vi "WriteConfiguration.vi"(8 "error in":errorcluster) -> (0 "error out":errorcluster)   [LabVIEW 2013]
uses:
  GlobalVariables/ValveParameters.vi
  <vilib>/Utility/config.llb/Write Key (U32).vi
  <vilib>/Utility/config.llb/Write Key (String).vi
  <vilib>/Utility/config.llb/Write Key (I32).vi
  GlobalVariables/CaptParameters.vi
  GlobalVariables/SystemParameters.vi
  GlobalVariables/PreconfiguredSleeveData.vi
  GlobalVariables/LanguagesSettings.vi
  <vilib>/Utility/config.llb/NI_LVConfig.lvlib
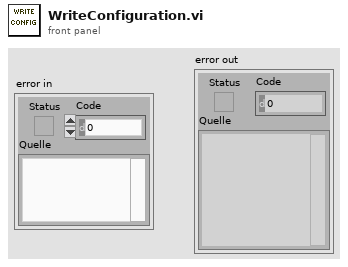
[diagram p1: front panel]
types:
  T1 = cluster{"baudrate":u32, "databits":u16, "paritybit":u16, "stopbits":u16, "flux control":u16, "Port":string, "Serial Parameters":cluster{"Mode":enum16{"RTU", "ASCII"}, "Slave Address":u8}, "Timeout":u32}
  T2 = typedef "NI_LVConfig.lvlib/Config Data RefNum.ctl" = refnum<k1>
  T3 = cluster{"baudrate":u32, "databits":u16, "paritybit":u16, "stopbits":u16, "flux control":u16, "Port":string, "Register Address":u16, "Serial Parameters":cluster{"Mode":enum16{"RTU", "ASCII"}, "Slave Address":u8}, "Timeout":u32}
  T4 = cluster{"defaultLanguage":string, "languageFile":string, "languages":string, "calibrationVolumeFile":string}
  T5 = cluster{"sleeveLength":dbl, "sleeveDiameter":dbl, "sleeveThickness":dbl}
  T6 = cluster{"SupportedLanguagesList":string[], "ActiveLanguage":string, "ActiveLanguageIndex":u16, "LocalisationFileContent[out]":cluster{"Indices":u32[], "LocalizedWords":string[][]}}
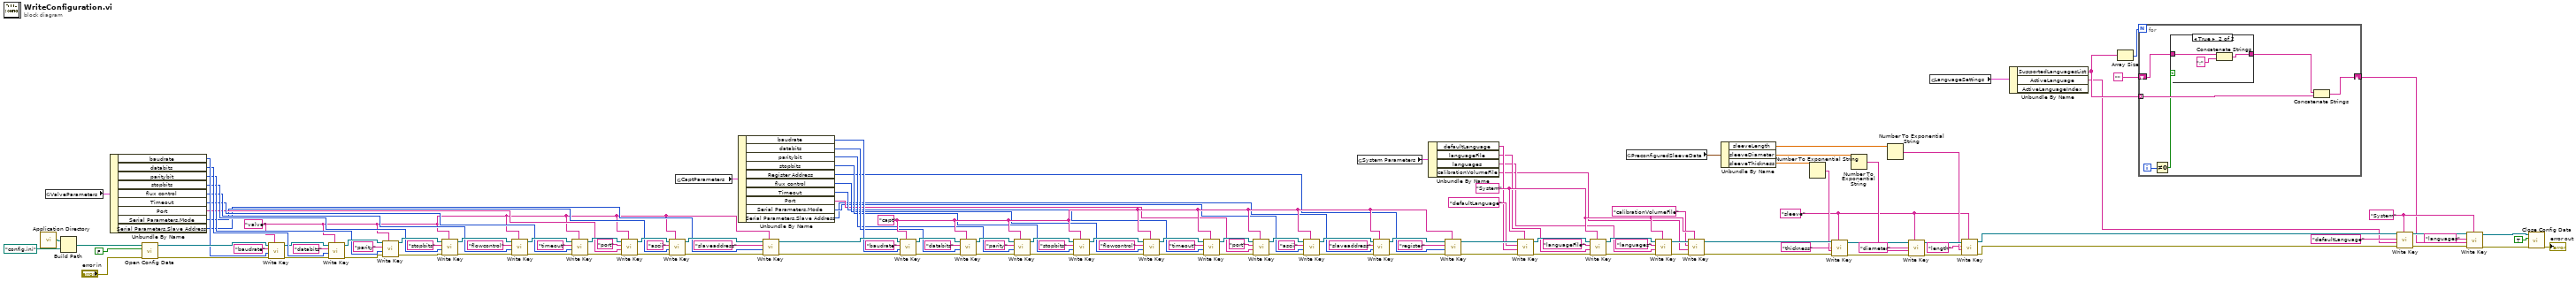
[diagram p0: block diagram]
diagram:
  w5 = "System"
  w19 = "sleeve"
  w41 = "System"
  w68 = "capt" ("section")
  w93 = "valve" ("section")
  n1 = call <vilib>:"Application Directory.vi"() -> ("Application Directory"=w130:path)
  n2 = global read "ValveParameters.vi" "ValveParameters"() -> (w127:T1)
  n3 = Build Path(base path=w130, name or relative path=path "config.ini" ("configuration file path")) -> (appended path=w128:path)
  n4 = Unbundle By Name(w127) -> ("baudrate"=w125:u32, "databits"=w122:u16, "paritybit"=w103:u16, "stopbits"=w102:u16, "flux control"=w101:u16, "Timeout"=w100:u32, "Port"=w99:string, "Serial Parameters.Mode"=w96:enum16{"RTU", "ASCII"}, "Serial Parameters.Slave Address"=w95:u8)
  n5 = call <vilib>:"Open Config Data.vi"("error in (no error)"="error in", "create file if necessary (T)"=FALSE ("create file if necessary? (T)"), "configuration file path"=w128) -> ("error out"=w137:errorcluster, "refnum"=w136:T2)  [unwired: 6 in, 1 out]
  n6 = call-poly <vilib>:"Write Key.vi"("section"=w93, "error in (no error)"=w137, "value"=w125, "key"="baudrate", "refnum"=w136) -> ("error out"=w134:errorcluster, "refnum out"=w121:T2)  [unwired: 4 in, 1 out]
  n7 = call-poly <vilib>:"Write Key.vi"("section"=w93, "error in (no error)"=w134, "value"=w122, "key"="databits", "refnum"=w121) -> ("error out"=w135:errorcluster, "refnum out"=w120:T2)  [unwired: 4 in, 1 out]
  n8 = call-poly <vilib>:"Write Key.vi"("section"=w93, "error in (no error)"=w135, "value"=w103, "key"="parity", "refnum"=w120) -> ("error out"=w114:errorcluster, "refnum out"=w119:T2)  [unwired: 4 in, 1 out]
  n9 = call-poly <vilib>:"Write Key.vi"("section"=w93, "error in (no error)"=w114, "value"=w102, "key"="stopbits", "refnum"=w119) -> ("error out"=w113:errorcluster, "refnum out"=w118:T2)  [unwired: 4 in, 1 out]
  n10 = call-poly <vilib>:"Write Key.vi"("section"=w93, "error in (no error)"=w113, "value"=w101, "key"="flowcontrol", "refnum"=w118) -> ("error out"=w112:errorcluster, "refnum out"=w117:T2)  [unwired: 4 in, 1 out]
  n11 = call-poly <vilib>:"Write Key.vi"("section"=w93, "error in (no error)"=w112, "value"=w100, "key"="timeout", "refnum"=w117) -> ("error out"=w111:errorcluster, "refnum out"=w116:T2)  [unwired: 4 in, 1 out]
  n12 = call-poly <vilib>:"Write Key.vi"("section"=w93, "error in (no error)"=w111, "value"=w99, "key"="port", "refnum"=w116) -> ("error out"=w110:errorcluster, "refnum out"=w115:T2)  [unwired: 4 in, 1 out]
  n13 = call-poly <vilib>:"Write Key.vi"("section"=w93, "error in (no error)"=w110, "value"=w96, "key"="ascii", "refnum"=w115) -> ("error out"=w109:errorcluster, "refnum out"=w108:T2)  [unwired: 4 in, 1 out]
  n14 = global read "CaptParameters.vi" "CaptParameters"() -> (w126:T3)
  n15 = Unbundle By Name(w126) -> ("baudrate"=w61:u32, "databits"=w60:u16, "paritybit"=w59:u16, "stopbits"=w58:u16, "Register Address"=w52:u16, "flux control"=w57:u16, "Timeout"=w56:u32, "Port"=w55:string, "Serial Parameters.Mode"=w54:enum16{"RTU", "ASCII"}, "Serial Parameters.Slave Address"=w53:u8)
  n16 = call-poly <vilib>:"Write Key.vi"("section"=w93, "error in (no error)"=w109, "value"=w95, "key"="slaveaddress", "refnum"=w108) -> ("error out"=w62:errorcluster, "refnum out"=w63:T2)  [unwired: 4 in, 1 out]
  n17 = call-poly <vilib>:"Write Key.vi"("section"=w68, "error in (no error)"=w62, "value"=w61, "key"="baudrate", "refnum"=w63) -> ("error out"=w91:errorcluster, "refnum out"=w88:T2)  [unwired: 4 in, 1 out]
  n18 = call-poly <vilib>:"Write Key.vi"("section"=w68, "error in (no error)"=w91, "value"=w60, "key"="databits", "refnum"=w88) -> ("error out"=w92:errorcluster, "refnum out"=w87:T2)  [unwired: 4 in, 1 out]
  n19 = call-poly <vilib>:"Write Key.vi"("section"=w68, "error in (no error)"=w92, "value"=w59, "key"="parity", "refnum"=w87) -> ("error out"=w81:errorcluster, "refnum out"=w86:T2)  [unwired: 4 in, 1 out]
  n20 = call-poly <vilib>:"Write Key.vi"("section"=w68, "error in (no error)"=w81, "value"=w58, "key"="stopbits", "refnum"=w86) -> ("error out"=w80:errorcluster, "refnum out"=w85:T2)  [unwired: 4 in, 1 out]
  n21 = call-poly <vilib>:"Write Key.vi"("section"=w68, "error in (no error)"=w80, "value"=w57, "key"="flowcontrol", "refnum"=w85) -> ("error out"=w79:errorcluster, "refnum out"=w84:T2)  [unwired: 4 in, 1 out]
  n22 = call-poly <vilib>:"Write Key.vi"("section"=w68, "error in (no error)"=w79, "value"=w56, "key"="timeout", "refnum"=w84) -> ("error out"=w78:errorcluster, "refnum out"=w83:T2)  [unwired: 4 in, 1 out]
  n23 = call-poly <vilib>:"Write Key.vi"("section"=w68, "error in (no error)"=w78, "value"=w55, "key"="port", "refnum"=w83) -> ("error out"=w77:errorcluster, "refnum out"=w82:T2)  [unwired: 4 in, 1 out]
  n24 = call-poly <vilib>:"Write Key.vi"("section"=w68, "error in (no error)"=w77, "value"=w54, "key"="ascii", "refnum"=w82) -> ("error out"=w76:errorcluster, "refnum out"=w75:T2)  [unwired: 4 in, 1 out]
  n25 = global read "SystemParameters.vi" "System Parameters"() -> (w50:T4)
  n26 = call-poly <vilib>:"Write Key.vi"("section"=w68, "error in (no error)"=w76, "value"=w53, "key"="slaveaddress", "refnum"=w75) -> ("error out"=w67:errorcluster, "refnum out"=w66:T2)  [unwired: 4 in, 1 out]
  n27 = Unbundle By Name(w50) -> ("defaultLanguage"=w39:string, "languageFile"=w38:string, "languages"=w35:string, "calibrationVolumeFile"=w34:string)
  n28 = call-poly <vilib>:"Write Key.vi"("section"=w68, "error in (no error)"=w67, "value"=w52, "key"="register", "refnum"=w66) -> ("error out"=w45:errorcluster, "refnum out"=w46:T2)  [unwired: 4 in, 1 out]
  n29 = call-poly <vilib>:"Write Key.vi"("section"=w41, "error in (no error)"=w45, "value"=w39, "key"="defaultLanguage", "refnum"=w46) -> ("error out"=w44:errorcluster, "refnum out"=w47:T2)  [unwired: 4 in, 1 out]
  n30 = call-poly <vilib>:"Write Key.vi"("section"=w41, "error in (no error)"=w44, "value"=w38, "key"="languageFile", "refnum"=w47) -> ("error out"=w43:errorcluster, "refnum out"=w48:T2)  [unwired: 4 in, 1 out]
  n31 = global read "PreconfiguredSleeveData.vi" "PreconfiguredSleeveData"() -> (w32:T5)
  n32 = call-poly <vilib>:"Write Key.vi"("section"=w41, "error in (no error)"=w43, "value"=w35, "key"="languages", "refnum"=w48) -> ("error out"=w42:errorcluster, "refnum out"=w49:T2)  [unwired: 4 in, 1 out]
  n33 = call-poly <vilib>:"Write Key.vi"("section"=w41, "error in (no error)"=w42, "value"=w34, "key"="calibrationVolumeFile", "refnum"=w49) -> ("error out"=w31:errorcluster, "refnum out"=w28:T2)  [unwired: 4 in, 1 out]
  n34 = Unbundle By Name(w32) -> ("sleeveLength"=w25:dbl, "sleeveDiameter"=w24:dbl, "sleeveThickness"=w23:dbl)
  n35 = Number To Exponential String(number=w23) -> (E-format string=w21:string)  [unwired: 3 in]
  n36 = call-poly <vilib>:"Write Key.vi"("section"=w19, "error in (no error)"=w31, "value"=w21, "key"="thickness", "refnum"=w28) -> ("error out"=w30:errorcluster, "refnum out"=w27:T2)  [unwired: 4 in, 1 out]
  n37 = Number To Exponential String(number=w24) -> (E-format string=w22:string)  [unwired: 3 in]
  n38 = Number To Exponential String(number=w25) -> (E-format string=w20:string)  [unwired: 3 in]
  n39 = call-poly <vilib>:"Write Key.vi"("section"=w19, "error in (no error)"=w30, "value"=w22, "key"="diameter", "refnum"=w27) -> ("error out"=w29:errorcluster, "refnum out"=w26:T2)  [unwired: 4 in, 1 out]
  n40 = global read "LanguagesSettings.vi" "LanguageSettings"() -> (w15:T6)
  n41 = call-poly <vilib>:"Write Key.vi"("section"=w19, "error in (no error)"=w29, "value"=w20, "key"="length", "refnum"=w26) -> ("error out"=w6:errorcluster, "refnum out"=w7:T2)  [unwired: 4 in, 1 out]
  n42 = Unbundle By Name(w15) -> ("SupportedLanguagesList"=w12:string[], "ActiveLanguage"=w3:string)  [unwired: 1 out]
  n43 = Array Size(array=w12) -> (size(s)=w14:i32)
  n44 = for {
    N: w14 -> [_]
    shift-right: [w140] -> w2
    shift-left: "" -> [w139]
    tunnel: w12 -> [w143] mode=indexing
    i -> [w141]
    n45 = Not Equal To 0?(x=w141) -> (x != 0?=w142:bool)
    n46 = case shown="True" w142 {
      tunnel: w139 -> [w144 w146]
      tunnel: [w144 w145] -> w138
      frame False {
      }
      frame True {
        n47 = Concatenate Strings(w146, ";") -> (w145:string)
      }
    }
    n48 = Concatenate Strings(w138, w143) -> (w140:string)
  }
  n49 = call-poly <vilib>:"Write Key.vi"("section"=w5, "error in (no error)"=w6, "value"=w3, "key"="defaultLanguage", "refnum"=w7) -> ("error out"=w8:errorcluster, "refnum out"=w9:T2)  [unwired: 4 in, 1 out]
  n50 = call-poly <vilib>:"Write Key.vi"("section"=w5, "error in (no error)"=w8, "value"=w2, "key"="languages", "refnum"=w9) -> ("error out"=w10:errorcluster, "refnum out"=w11:T2)  [unwired: 4 in, 1 out]
  n51 = call <vilib>:"Close Config Data.vi"("error in (no error)"=w10, "write file if changed (T)"=TRUE ("create file if necessary? (T)"), "refnum"=w11) -> ("error out"=→"error out":errorcluster)  [unwired: 7 in, 1 out]
